vi "Create DIDPID HardwareInput Signal.vi"(8 "error in (no error)":errorcluster, 10 "Signal Parameters":T2 {"Byte Order" items=["Little Endian", "Big Endian"]; "Data Type" items=["Signed", "Unsigned", "IEEE Float"]}, 11 "Section Ptr":T1 format="%.0x") -> (0 "error out":errorcluster, 3 "Section Ptr out":T1 format="%.0x")   [LabVIEW 2015, in "Diagnostics Addon Shared.lvlib"]
uses:
  Diagnostics Addon Shared.lvlib
  DIDPID Signal Parameters.ctl
  <vilib>/NI Veristand/Custom Device API/Custom Device Item Ref.ctl
  <vilib>/NI Veristand/Custom Device API/Custom Device Channel.ctl
  <vilib>/NI Veristand/Custom Device API/Custom Device Channel Type.ctl
  GUID Lookup.vi
  <vilib>/NI Veristand/Custom Device API/Custom Device API.lvlib
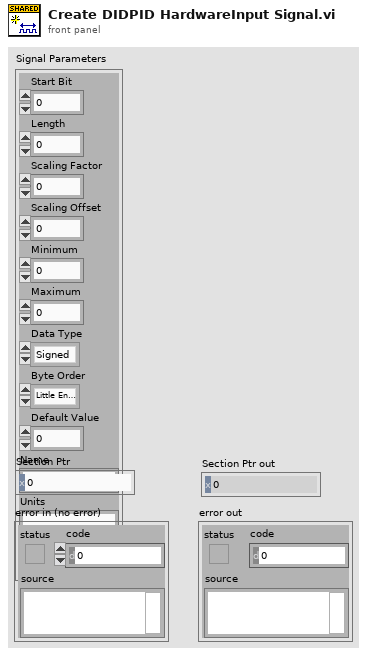
[diagram p1: front panel]
types:
  T1 = typedef "Custom Device API.lvlib/Custom Device Item Ref.ctl" = u64
  T2 = typedef "Diagnostics Addon Shared.lvlib/DIDPID Signal Parameters.ctl" = cluster{"Start Bit":u8, "Length":u8, "Scaling Factor":dbl, "Scaling Offset":dbl, "Minimum":dbl, "Maximum":dbl, "Data Type":u32, "Byte Order":u32, "Default Value":dbl, "Name":string, "Units":string, "Description":string}
  T3 = typedef "Custom Device API.lvlib/Custom Device Channel.ctl" = cluster{"Type":T4, "Units":string, "Default Value":dbl, "Faultable":bool, "Scalable":bool}
  T4 = typedef "Custom Device API.lvlib/Custom Device Channel Type.ctl" = enum16{"Input", "Output"}
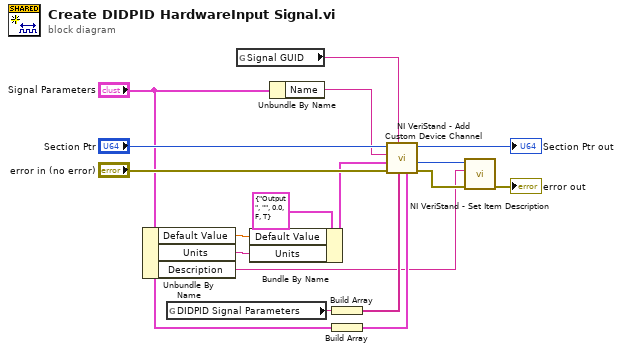
[diagram p0: block diagram]
diagram:
  n1 = Unbundle By Name("Signal Parameters") -> ("Default Value"=w5:dbl, "Units"=w4:string, "Description"=w1:string)
  n2 = global read "GUID Lookup.vi" "DIDPID Signal Parameters"() -> (w15:string)
  n3 = global read "GUID Lookup.vi" "Signal GUID"() -> (w10:string)
  n4 = Bundle By Name(cluster=T3 {"Type"=enum."Output", "Units"="", "Default Value"=0.0, "Faultable"=FALSE, "Scalable"=TRUE} ("Channel"), "Default Value"=w5, "Units"=w4) -> (w2:T3)
  n5 = Unbundle By Name("Signal Parameters") -> ("Name"=w13:string)
  n6 = Build Array(w15) -> (w16:string[])
  n7 = Build Array("Signal Parameters") -> (w14:T2[])
  n8 = call <vilib>:"NI VeriStand - Add Custom Device Channel.vi"("Property Values"=w14, "Property names"=w16, "GUID (Default Channel)"=w10, "error in (no error)"="error in (no error)", "Channel"=w2, "Channel Name"=w13, "Parent Ref in"="Section Ptr") -> ("error out"=w8:errorcluster, "Channel Ref"=w9:T1, "Parent Ref out"=→"Section Ptr out":T1)  [unwired: 1 in, 1 out]
  n9 = call <vilib>:"NI VeriStand - Set Item Description.vi"("error in (no error)"=w8, "Description"=w1, "Item Ref in"=w9) -> ("error out"=→"error out":errorcluster)  [unwired: 6 in, 2 out]
